vi "Relay Control.vi"() -> ()   [LabVIEW 2013]
uses:
  <vilib>/Instr/_visa.llb/VISA Configure Serial Port (Instr).vi
panel:
  in  "Bytes at Port":u32
  in  "Addr":u8
  out "return count":u32
  out "unsigned byte array 2":u8[](array[numeric]) format="%08b"
  out "x .xor. y?":u8
  in  "wait 2":u32
  in  "baud rate (9600)":u32=19200
  out "unsigned byte array":u8[](array[numeric]) format="%08b"
  in  "wait":u32
  out "read buffer":string
  out "resulting string":string
  in  "stop":bool
  in  "Data":u8 format="%b"
  in  "Command":u8
  in  "SET":bool
  in  "VISA resource name":refnum<visa-resource-name>
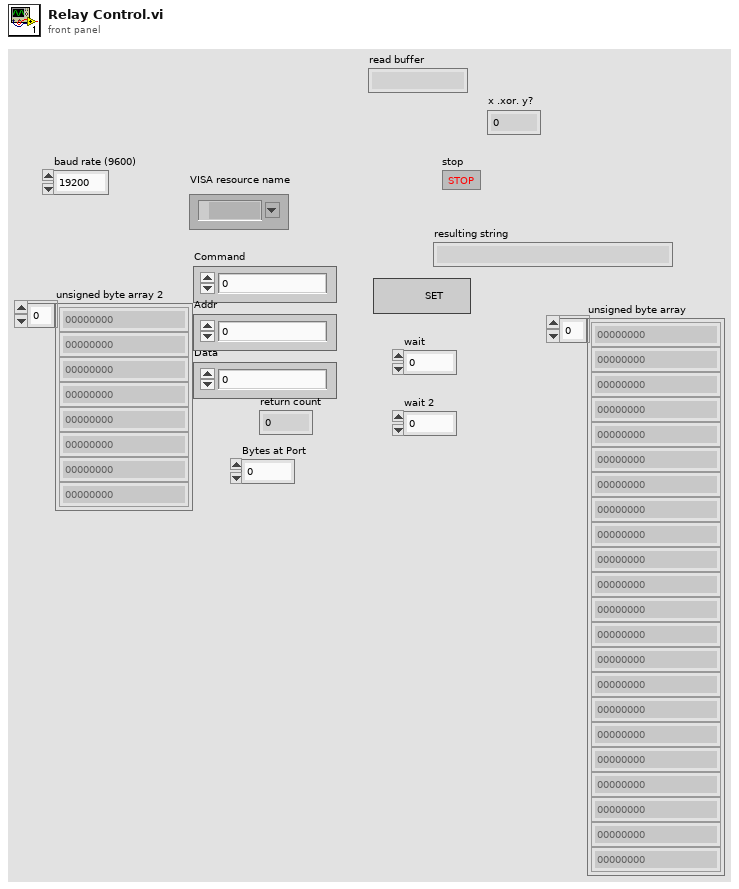
[diagram p1: front panel]
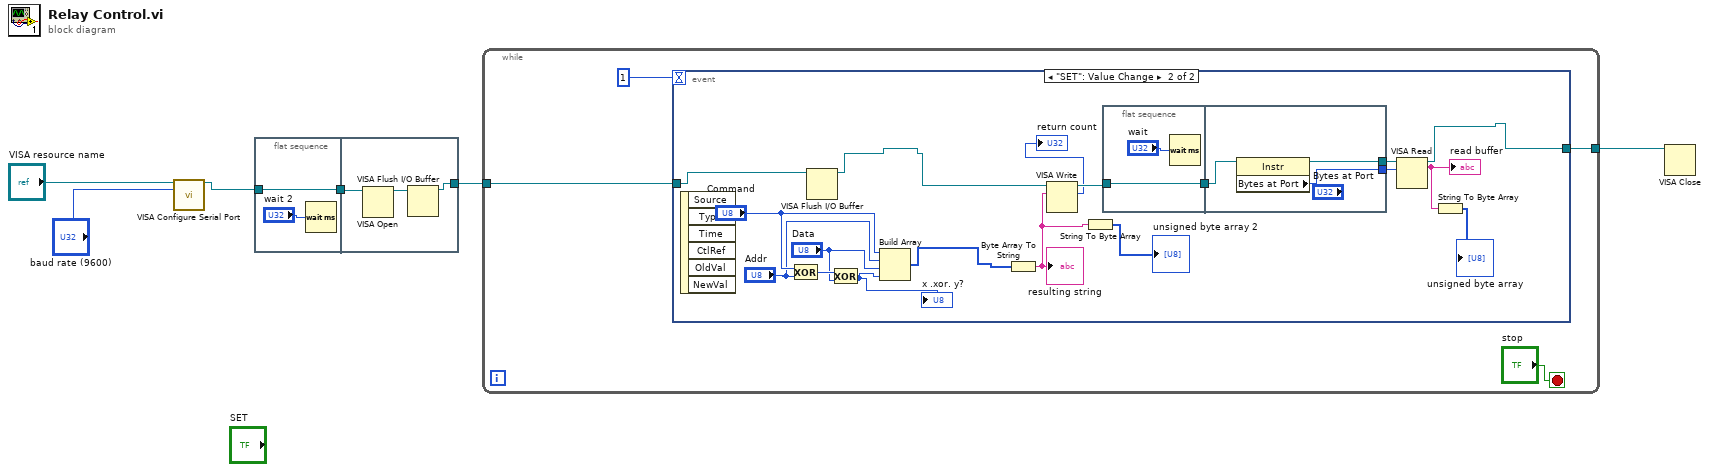
[diagram p0: block diagram]
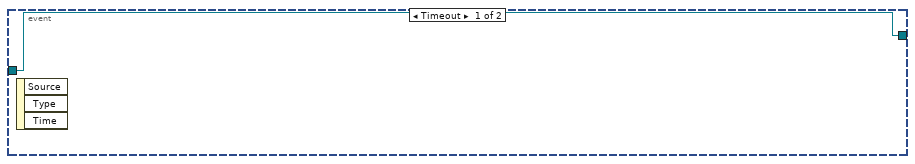
[diagram p2: hidden frame]
diagram:
  n1 = call-poly "VISA Configure Serial Port"("VISA resource name"="VISA resource name", "baud rate (9600)"="baud rate (9600)") -> ("VISA resource name out"=w1:refnum<visa-resource-name>)  [unwired: 12 in, 1 out]
  n2 = flat-sequence {
    tunnel: w1 -> [w8]
    tunnel: [w8] -> w3
    tunnel: [w11] -> w4
    tunnel: w3 -> [w10]
    frame #0 {
      n3 = Wait (ms)(milliseconds to wait="wait 2") -> ()  [unwired: 1 out]
    }
    frame #1 {
      n4 = VISA Open(VISA resource name=w10) -> (VISA resource name=w9:refnum<visa-resource-name>)  [unwired: 4 in, 1 out]
      n5 = VISA Flush I/O Buffer(VISA resource name=w9) -> (VISA resource name out=w11:refnum<visa-resource-name>)  [unwired: 2 in, 1 out]
    }
  }
  n6 = while {
    tunnel: w4 -> [w13]
    tunnel: [w12] -> w2
    stop <- "stop" stop-if-true
    n7 = event shown="[1] \"SET\": Value Change" {
      selector: _ -> [_ _]
      dyn-events: _ -> [_ _]
      timeout: 1 -> [_ _]
      tunnel: w13 -> [w16 w20]
      tunnel: [w16 w17] -> w12
      event Timeout {
        n8 = event-data() -> ()  [unwired: 1 in, 3 out]
      }
      event "SET": Value Change {
        n9 = event-data() -> ()  [unwired: 1 in, 6 out]
        n10 = Exclusive Or(1:"Addr", 2:"Command") -> (0:w34:u8)
        n11 = VISA Flush I/O Buffer(VISA resource name=w20) -> (VISA resource name out=w18:refnum<visa-resource-name>)  [unwired: 2 in, 1 out]
        n12 = Exclusive Or(1:"Data", 2:w34) -> (0:w24:u8)
        "x .xor. y?" <- w24
        n13 = Build Array("Command", "Addr", "Data", w24) -> (w27:u8[])
        n14 = Byte Array To String(unsigned byte array=w27) -> (string=w26:string)
        "resulting string" <- w26
        n15 = VISA Write(VISA resource name=w18, write buffer=w26) -> (VISA resource name out=w23:refnum<visa-resource-name>, return count=→"return count":u32)  [unwired: 1 in, 1 out]
        n16 = String To Byte Array(string=w26) -> (unsigned byte array=→"unsigned byte array 2":u8[])
        n17 = flat-sequence {
          tunnel: w23 -> [w35]
          tunnel: [w35] -> w30
          tunnel: [w39] -> w31
          tunnel: w30 -> [w38]
          tunnel: [w37] -> w19
          frame #0 {
            n18 = Wait (ms)(milliseconds to wait="wait") -> ()  [unwired: 1 out]
          }
          frame #1 {
            n19 = property class="Instr"(reference=w38) -> (reference out=w39:refnum<visa-resource-name>, "Bytes at Port"=w37:u32)  [unwired: 1 in, 1 out]
          }
        }
        n20 = VISA Read(VISA resource name=w31, byte count=w19) -> (VISA resource name out=w17:refnum<visa-resource-name>, read buffer=w29:string)  [unwired: 1 in, 2 out]
        "read buffer" <- w29
        n21 = String To Byte Array(string=w29) -> (unsigned byte array=→"unsigned byte array":u8[])
      }
    }
  }
  n22 = VISA Close(VISA resource name=w2) -> ()  [unwired: 1 in, 1 out]
